vi "case_structures.vi"() -> ()   [LabVIEW 2014]
panel:
  out "Result 2":string
  in  "State":T1(ring)
  out "Result":string
  in  "True/False":bool
  # "Binary State"
  # "Enumerated State"
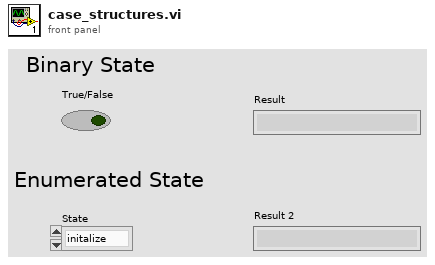
[diagram p1: front panel]
types:
  T1 = enum16{"initalize", "wait", "execute", "terminate"}
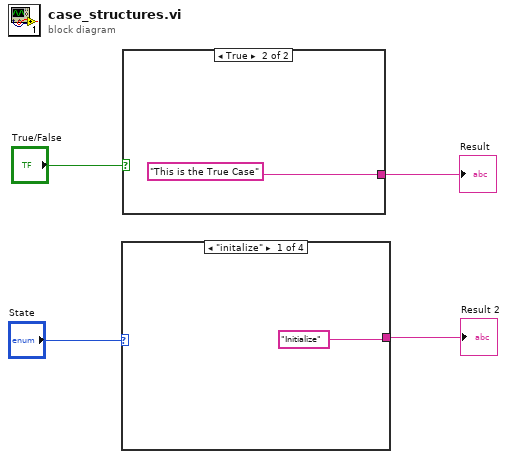
[diagram p0: block diagram]
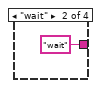
[diagram p2: hidden frame]
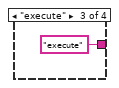
[diagram p3: hidden frame]
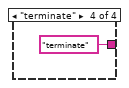
[diagram p4: hidden frame]
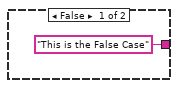
[diagram p5: hidden frame]
diagram:
  n1 = case shown="\"initalize\"" "State" {
    tunnel: ["Initialize" ("Result") "wait" ("Result") "execute" ("Result") "terminate" ("Result")] -> w1
    frame "initalize" {
    }
    frame "wait" {
    }
    frame "execute" {
    }
    frame "terminate" {
    }
  }
  "Result 2" <- w1
  n2 = case shown="True" "True/False" {
    tunnel: ["This is the False Case" ("Result") "This is the True Case" ("Result")] -> w3
    frame False {
    }
    frame True {
    }
  }
  "Result" <- w3
